vi "createPublishString.vi"(8 "error in (no error)":errorcluster, 9 "parameter":string, 10 "publishers":T1, 11 "MonoCommunicator in":refnum<class "MonoCommunicator.lvclass">) -> (0 "error out":errorcluster, 2 "string":string, 3 "MonoCommunicator out":refnum<class "MonoCommunicator.lvclass">)   [LabVIEW 2016, in "MonoCommunicator.lvclass"]
uses:
  MonoCommunicator.lvclass
  Typedefs/publishers.ctl
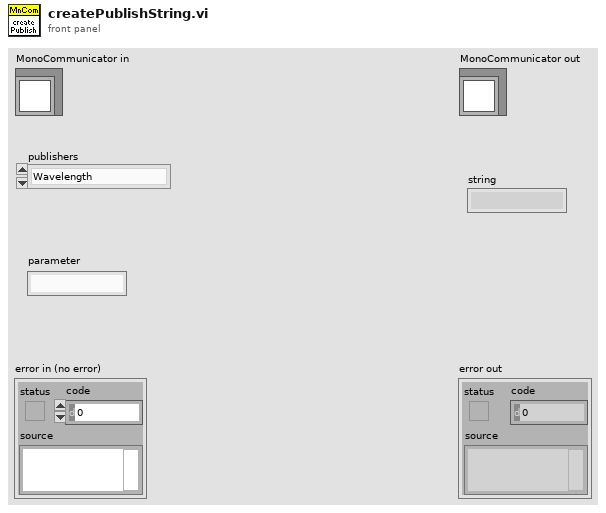
[diagram p1: front panel]
types:
  T1 = typedef "publishers.ctl" = enum16{"Wavelength", "Grating", "FrontEntranceSlitPosition", "FrontExitSlitPosition", "SoftwareStatus", "MonochromatorId"}
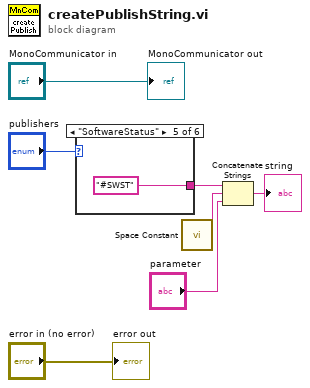
[diagram p0: block diagram]
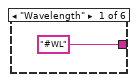
[diagram p2: hidden frame]
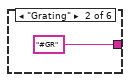
[diagram p3: hidden frame]
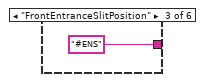
[diagram p4: hidden frame]
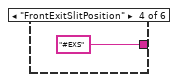
[diagram p5: hidden frame]
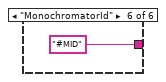
[diagram p6: hidden frame]
diagram:
  n1 = case shown="\"SoftwareStatus\"" "publishers" {
    tunnel: ["#WL" ("string") "#GR" ("string") "#ENS" ("string") "#EXS" ("string") "#SWST" ("string") "#MID" ("string")] -> w1
    frame "Wavelength" {
    }
    frame "Grating" {
    }
    frame "FrontEntranceSlitPosition" {
    }
    frame "FrontExitSlitPosition" {
    }
    frame "SoftwareStatus" {
    }
    frame "MonochromatorId" {
    }
  }
  n2 = call <vilib>:"Space Constant.vi"() -> ("String"=w6:string)
  n3 = Concatenate Strings(w1, w6, "parameter") -> (→"string":string)
  "error out" <- "error in (no error)"
  "MonoCommunicator out" <- "MonoCommunicator in"
